vi "Append and Prepend String to filename.vi"(0 "Prepend String":string, 2 "Original file path":path, 5 "Append String":string) -> (16 "New file path":path)   [LabVIEW 2022 SP3, in "Generic Utilities.lvclass"]
uses:
  Generic Utilities.lvclass
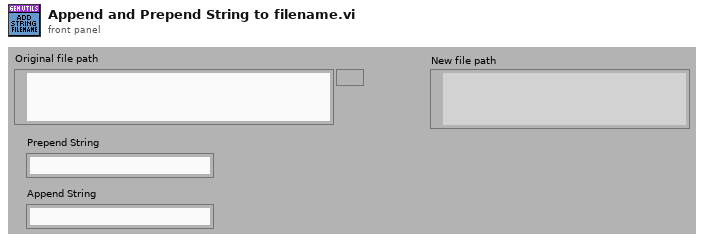
[diagram p1: front panel]
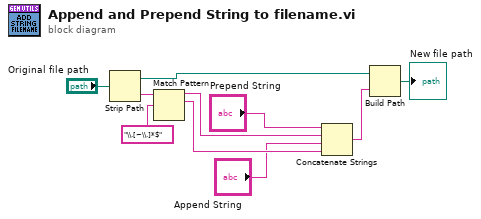
[diagram p0: block diagram]
diagram:
  n1 = Strip Path(path="Original file path") -> (stripped path=w5:path, name=w9:string)
  n2 = Match Pattern(string=w9, regular expression="\\.[~\\.]*$") -> (before substring=w6:string, match substring=w7:string)  [unwired: 3 out]
  n3 = Concatenate Strings("Prepend String", w6, "Append String", w7) -> (w4:string)
  n4 = Build Path(base path=w5, name or relative path=w4) -> (appended path=→"New file path":path)
